vi "未命名 1.vi"() -> ()   [LabVIEW 2022 SP3]
panel:
  out "无符号字节数组":u8[](array[numeric])
  out "处理后的字符串":string
  out "波形图":waveform(dbl)(graph)
  out "t 时间分量":dbl
  out "Y INC":dbl
  out "Y REF":dbl
  out "Y OFF":dbl
  in  "停止":bool
  out "data":string
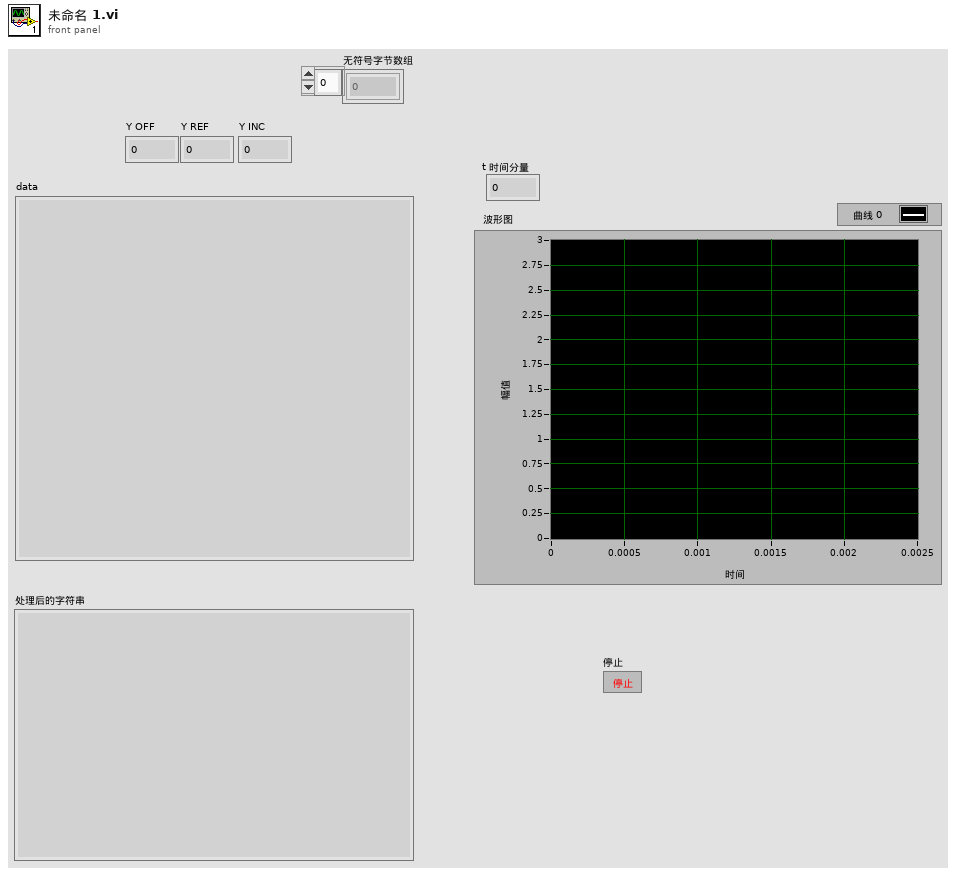
[diagram p1: front panel]
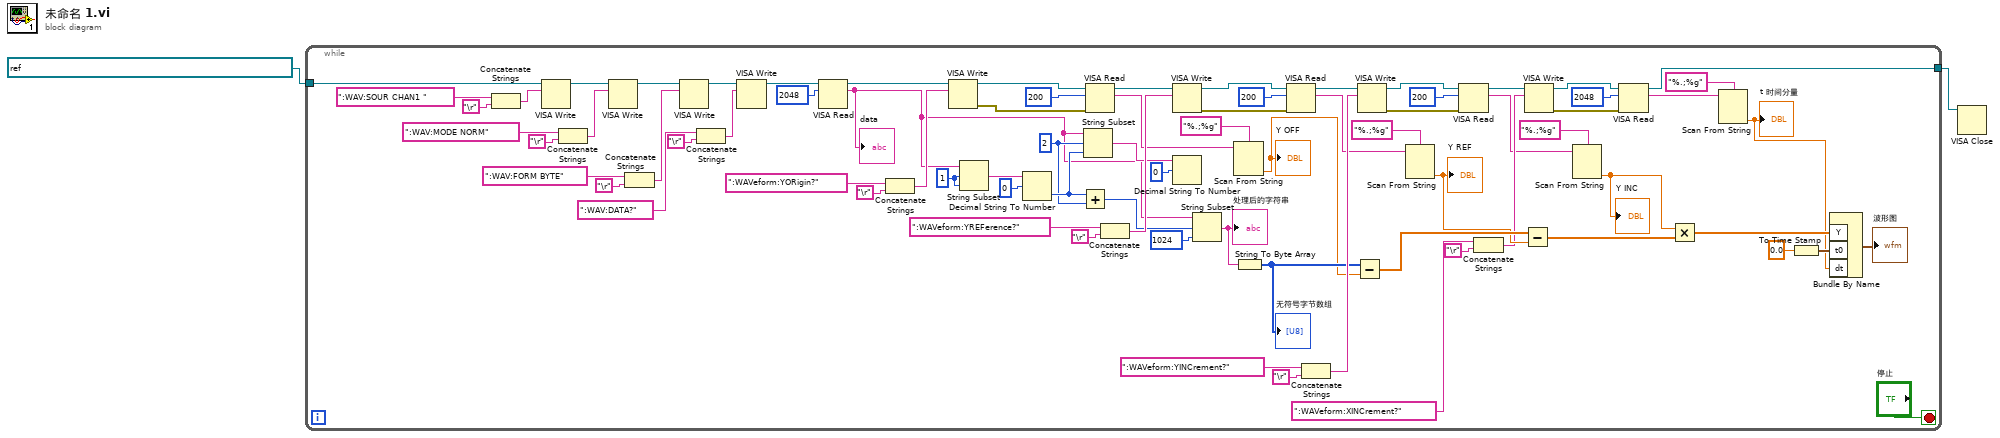
[diagram p0: block diagram]
diagram:
  n1 = while {
    tunnel: refnum<visa-resource-name> "USB0::0x1AB1::0x0517::DS1ZE251002707::INSTR" ("引用") -> [w66]
    tunnel: [w9] -> w2
    stop <- "停止" stop-if-true
    w36 = 2 ("长度（剩余）")
    w42 = 1 ("偏移量(0)")
    n2 = Concatenate Strings(":WAV:SOUR CHAN1 ", "\r") -> (w73:string)
    n3 = VISA Write(VISA resource name=w66, write buffer=w73) -> (VISA resource name out=w65:refnum<visa-resource-name>)  [unwired: 1 in, 2 out]
    n4 = Concatenate Strings(":WAV:MODE NORM", "\r") -> (w70:string)
    n5 = VISA Write(VISA resource name=w65, write buffer=w70) -> (VISA resource name out=w64:refnum<visa-resource-name>)  [unwired: 1 in, 2 out]
    n6 = Concatenate Strings(":WAV:FORM BYTE", "\r") -> (w67:string)
    n7 = VISA Write(VISA resource name=w64, write buffer=w67) -> (VISA resource name out=w63:refnum<visa-resource-name>)  [unwired: 1 in, 2 out]
    n8 = Concatenate Strings(":WAV:DATA?", "\r") -> (w77:string)
    n9 = VISA Write(VISA resource name=w63, write buffer=w77) -> (VISA resource name out=w14:refnum<visa-resource-name>)  [unwired: 1 in, 2 out]
    n10 = VISA Read(VISA resource name=w14, byte count=u32 2048 ("字节总数")) -> (VISA resource name out=w13:refnum<visa-resource-name>, read buffer=w29:string)  [unwired: 1 in, 2 out]
    "data" <- w29
    n11 = Concatenate Strings(":WAVeform:YORigin?" ("写入缓冲区"), "\r") -> (w57:string)
    n12 = VISA Write(VISA resource name=w13, write buffer=w57) -> (VISA resource name out=w61:refnum<visa-resource-name>, error out=w62:errorcluster)  [unwired: 1 in, 1 out]
    n13 = String Subset(string=w29, offset (0)=w42, length (rest)=w42) -> (substring=w40:string)
    n14 = Decimal String To Number(string=w40, offset=0 ("偏移量")) -> (number=w37:i32)  [unwired: 1 in, 1 out]
    n15 = Add(x=w37, y=w36) -> (x+y=w30:i32)
    n16 = String Subset(string=w29, offset (0)=w36, length (rest)=w37) -> (substring=w38:string)
    n17 = VISA Read(VISA resource name=w61, byte count=u32 200 ("字节总数"), error in (no error)=w62) -> (VISA resource name out=w50:refnum<visa-resource-name>, read buffer=w34:string)  [unwired: 2 out]
    n18 = Concatenate Strings(":WAVeform:YREFerence?" ("写入缓冲区"), "\r") -> (w51:string)
    n19 = VISA Write(VISA resource name=w50, write buffer=w51) -> (VISA resource name out=w55:refnum<visa-resource-name>, error out=w56:errorcluster)  [unwired: 1 in, 1 out]
    n20 = Decimal String To Number(string=w38, offset=0 ("偏移量")) -> ()  [unwired: 1 in, 2 out]
    n21 = String Subset(string=w29, offset (0)=w30, length (rest)=1024 ("长度（剩余）")) -> (substring=w27:string)
    "处理后的字符串" <- w27
    n22 = Scan From String(format string="%.;%g" ("格式字符串"), input string=w34) -> (output 1=w25:dbl)  [unwired: 3 in, 3 out]
    "Y OFF" <- w25
    n23 = String To Byte Array(string=w27) -> (unsigned byte array=w26:u8[])
    "无符号字节数组" <- w26
    n24 = VISA Read(VISA resource name=w55, byte count=u32 200 ("字节总数"), error in (no error)=w56) -> (VISA resource name out=w43:refnum<visa-resource-name>, read buffer=w31:string)  [unwired: 2 out]
    n25 = Concatenate Strings(":WAVeform:YINCrement?" ("写入缓冲区"), "\r") -> (w44:string)
    n26 = Subtract(x=w26, y=w25) -> (x-y=w24:dbl[])
    n27 = VISA Write(VISA resource name=w43, write buffer=w44) -> (VISA resource name out=w48:refnum<visa-resource-name>, error out=w49:errorcluster)  [unwired: 1 in, 1 out]
    n28 = Scan From String(format string="%.;%g" ("格式字符串"), input string=w31) -> (output 1=w23:dbl)  [unwired: 3 in, 3 out]
    "Y REF" <- w23
    n29 = VISA Read(VISA resource name=w48, byte count=u32 200 ("字节总数"), error in (no error)=w49) -> (VISA resource name out=w10:refnum<visa-resource-name>, read buffer=w4:string)  [unwired: 2 out]
    n30 = Concatenate Strings(":WAVeform:XINCrement?" ("写入缓冲区"), "\r") -> (w15:string)
    n31 = Subtract(x=w24, y=w23) -> (x-y=w21:dbl[])
    n32 = VISA Write(VISA resource name=w10, write buffer=w15) -> (VISA resource name out=w19:refnum<visa-resource-name>, error out=w20:errorcluster)  [unwired: 1 in, 1 out]
    n33 = Scan From String(format string="%.;%g" ("格式字符串"), input string=w4) -> (output 1=w22:dbl)  [unwired: 3 in, 3 out]
    "Y INC" <- w22
    n34 = VISA Read(VISA resource name=w19, byte count=u32 2048 ("字节总数"), error in (no error)=w20) -> (VISA resource name out=w9:refnum<visa-resource-name>, read buffer=w11:string)  [unwired: 2 out]
    n35 = Multiply(x=w22, y=w21) -> (x*y=w8:dbl[])
    n36 = Scan From String(format string="%.;%g" ("格式字符串"), input string=w11) -> (output 1=w5:dbl)  [unwired: 3 in, 3 out]
    "t 时间分量" <- w5
    n37 = To Time Stamp(1:0.0 ("数字")) -> (0:w6:timestamp)
    n38 = Bundle By Name("Y"=w8, "t0"=w6, "dt"=w5) -> (→"波形图":waveform(dbl))  [unwired: 1 in]
  }
  n39 = VISA Close(VISA resource name=w2) -> ()  [unwired: 1 in, 1 out]
